vi "Autonomous.vi"() -> ()   [LabVIEW 2018]
doc: "This VI starts when autonomous period begins, and will automatically be terminated when it ends. You can carry out timed or sensor driven operations directly to I/O or to subsystems without needing to return to the caller."
uses:
  Framework/Robot Global Data.vi
panel:
  in  "AutoFileName (with extension) (replace with dashboard selectors)":string="test.txt"
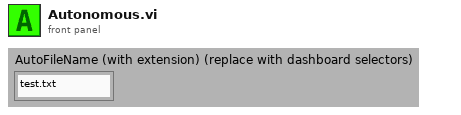
[diagram p1: front panel]
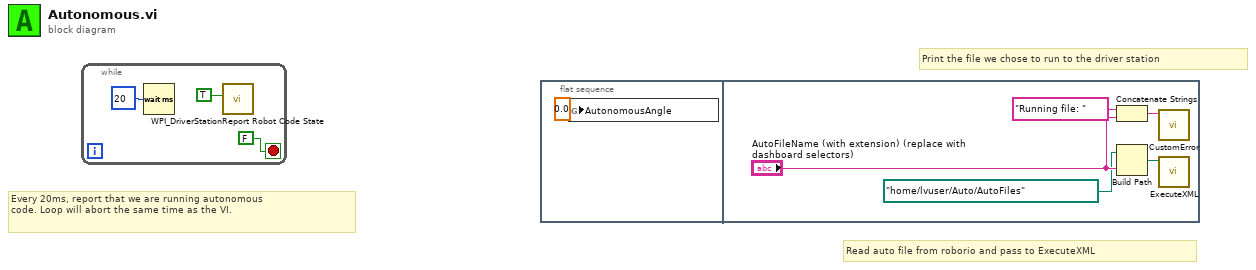
[diagram p0: block diagram]
diagram:
  # "Print the file we chose to run to the driver station"
  # "Read auto file from roborio and pass to ExecuteXML"
  # "Every 20ms, report that we are running autonomous\ncode. Loop will abort the same time as the VI."
  n1 = while {
    stop <- FALSE stop-if-true
    n2 = Wait (ms)(milliseconds to wait=u32 20) -> ()  [unwired: 1 out]
    n3 = call <vilib>:"WPI_DriverStationReport Robot Code State.vi"("Autonomous"=TRUE) -> ()  [unwired: 10 in, 1 out]
  }
  n4 = flat-sequence {
    frame #0 {
      n5 = global write "Robot Global Data.vi" "AutonomousAngle"(0.0 ("AutonomousAngle")) -> ()
    }
    frame #1 {
      n6 = Concatenate Strings("Running file: " ("string"), "AutoFileName (with extension) (replace with dashboard selectors)") -> (w9:string)
      n7 = Build Path(base path=path "/home/lvuser/Auto/AutoFiles", name or relative path="AutoFileName (with extension) (replace with dashboard selectors)") -> (appended path=w7:path)
      n8 = call "CustomError.vi"("String"=w9) -> ()  [unwired: 10 in, 1 out]
      n9 = call "ExecuteXML.vi"("Auto File Path"=w7) -> ()  [unwired: 10 in, 1 out]
    }
  }
